vi "Blank_string.vi"(11 "String I/P":string) -> (3 "Boolean":bool)   [LabVIEW 2017]
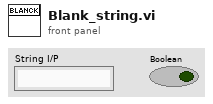
[diagram p1: front panel]
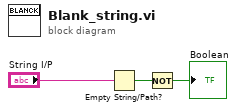
[diagram p0: block diagram]
diagram:
  n1 = Empty String/Path?(string/path="String I/P") -> (empty?=w2:bool)
  n2 = Not(x=w2) -> (.not. x?=→"Boolean":bool)
